vi "Assert Panel.vi"   [LabVIEW 2015]
uses:
  Models/PanelManager/PanelManager.lvclass
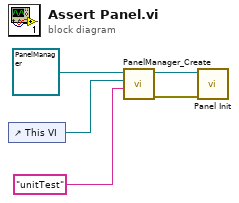
[diagram p0: block diagram]
diagram:
  n1 = control-ref of="This VI"() -> (w4:refnum<vi>)
  n2 = call "PanelManager_Create.vi"("Panel Name"="unitTest", "VI Refnum"=w4, "PanelManager in"=refnum<class "PanelManager.lvclass"> refnum ("PanelManager.lvclass")) -> ("error out"=w3:errorcluster, "PanelManager out"=w2:refnum<class "PanelManager.lvclass">)  [unwired: 7 in]
  n3 = call "Panel Init.vi"("error in (no error)"=w3, "PanelManager in"=w2) -> ()  [unwired: 8 in, 2 out]
